vi "Stop Wrapper.vi"(10 "final error code":i32, 11 "gController in":refnum<class "gController.lvclass">) -> ()   [LabVIEW 2017, in "Controller.lvlib" / "gController.lvclass"]
uses:
  gController.lvclass
  Session/Raw FPGA/FPGA Session.lvclass
  C:/Program Files (x86)/National Instruments/LabVIEW 2017/vi.lib/MSR Consulting, LLC/General Reuse/Session APIs/_Session Fwk/Session - Root.lvclass
  gController.lvclass/gController.ctl
  Data/SOAP Data.lvclass/SOAP Data.ctl
  Data/Read message_data.vi
  <vilib>/MSR Consulting, LLC/General Reuse/Session APIs/_Session Fwk/Session - Root.lvclass
  Data/SOAP Data.lvclass
panel:
  out "final error code 2":i32
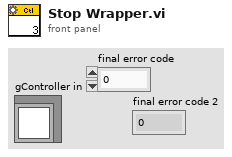
[diagram p1: front panel]
types:
  T1 = typedef "Session - Root.lvclass/Session Handle.ctl" = refnum<data-value>
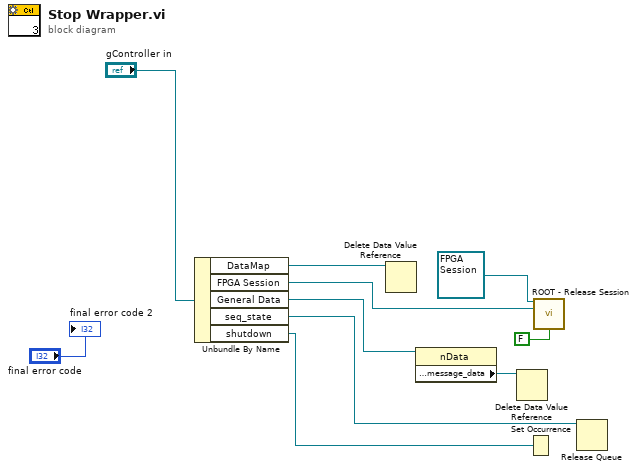
[diagram p0: block diagram]
diagram:
  n1 = Unbundle By Name("gController in") -> ("DataMap"=w3:refnum<data-value>, "FPGA Session"=w4:T1, "General Data"=w7:refnum<class "SOAP Data.lvclass">, "seq_state"=w9:refnum<queue>, "shutdown"=w10:refnum<k4>)
  n2 = Delete Data Value Reference(data value reference=w3) -> ()  [unwired: 1 in, 2 out]
  n3 = property class="nData"(reference=w7) -> ("Accessors:message_data"=w8:refnum<data-value>)  [unwired: 1 in, 2 out]
  n4 = Delete Data Value Reference(data value reference=w8) -> ()  [unwired: 1 in, 2 out]
  n5 = Set Occurrence(w10) -> ()
  n6 = call <vilib>:"ROOT - Release Session.vi"("OBJ - Session in"=refnum<class "FPGA Session.lvclass"> refnum ("FPGA Session"), "Session Handle in"=w4, "force destroy? (F)"=FALSE) -> ()  [unwired: 11 in, 2 out]
  n7 = Release Queue(queue=w9) -> ()  [unwired: 2 in, 3 out]
  "final error code 2" <- "final error code"
